vi "FaceDistances.vi"(8 "error in (no error)":errorcluster, 9 "faceToCompare":refnum<k24>, 10 "faceEncodings":refnum<k24>, 11 "FaceRecognition in":refnum<class "FaceRecognition.lvclass">) -> (0 "error out":errorcluster, 1 "FaceDistances":refnum<k24>, 3 "FaceRecognition out":refnum<class "FaceRecognition.lvclass">)   [LabVIEW 2020, in "FaceRecognitionDotNet.lvlib" / "FaceRecognition.lvclass"]
uses:
  FaceRecognition.lvclass
  dll/FaceRecognitionDotNet.dll
  FaceRecognition.lvclass/FaceRecognition.ctl
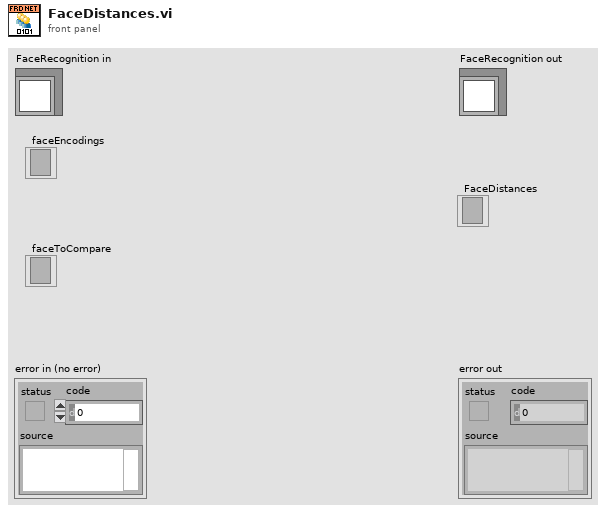
[diagram p1: front panel]
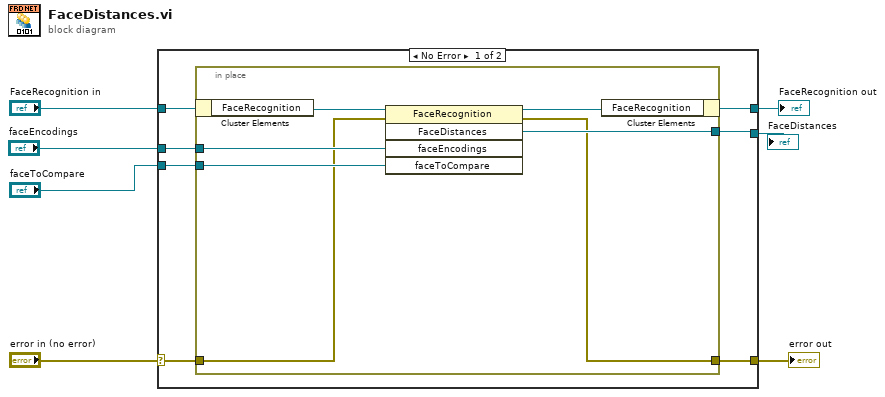
[diagram p0: block diagram]
diagram:
  n1 = case shown="No Error" "error in (no error)" {
    selector: "error in (no error)" -> [w12 w23]
    tunnel: [w11 w23] -> w6
    tunnel: [w13 w22] -> w4
    tunnel: "FaceRecognition in" -> [w14 w22]
    tunnel: [w10 _] -> w1
    tunnel: "faceToCompare" -> [w9 _]
    tunnel: "faceEncodings" -> [w8 _]
    frame No Error {
      n2 = in-place {
        in-place-border: w12 -> [w16]
        in-place-border: [w15] -> w11
        in-place-border: [w19] -> w10
        in-place-border: w9 -> [w18]
        in-place-border: w8 -> [w17]
        n3 = in-place-cluster #1(w14) -> ("FaceRecognition"=w21:refnum<k24>)
        n4 = invoke class="FaceRecognition" method="FaceDistances"(reference=w21, error in=w16, "faceEncodings"=w17, "faceToCompare"=w18) -> (reference out=w20:refnum<k24>, error out=w15:errorcluster, "FaceDistances"=w19:refnum<k24>)  [unwired: 1 in, 2 out]
        n5 = in-place-cluster #1("FaceRecognition"=w20) -> (w13:refnum<class "FaceRecognition.lvclass">)
      }
    }
    frame Error {
    }
  }
  "error out" <- w6
  "FaceRecognition out" <- w4
  "FaceDistances" <- w1
